vi "GoToKick.vi"(1 "goleiro?":bool, 3 "balls":T3[](array[typedef]), 4 "Robot in in":T4, 5 "atacando contra?":bool, 6 "Field Size in":T2, 7 "Target":dbl[](array[numeric]), 8 "Defender":bool, 9 "D ball - robot":dbl, 10 "AI Parameters":T1={"GotoKick"={"Dist do cone a frente"=150.0, "attacker farback"=1500.0, "Perto"=300.0, "min dist to kick"=150.0, "kick eps"=0.05, "Time to transition"=0.0}, "Attacker"={"CC chute"=0.09, "CC passe"=0.045, "Kick Force"=100.0, "D ball-robot Kick"=200.0, "D ball-robot Pass"=0.3}, "Defender"={"D max"=1700.0, "Vel p/ robô av"=1000.0, "Kick Force"=100.0, "D atk-def"=0.0, "D farback"=0.0}, "Timeout"={"Field/v in x"=6.0, "Dist Robots"=300, "Dist up in y"=300}, "Pose Striker"={"dist"=200.0, "Numeric"=-4.0, "dist 2"=200.0}, "Dist Stop"=300.0, "Distance when ball out"=200, "D central gap "=150.0, "T pass"=0.0, "Force ++"=0.0, "range kick"=0.0, "Chute alto"=TRUE, "Marcador novo"=TRUE} {"D central gap" format="%#_13g"; "Dist Stop" format="%#_13g"; "Pose Striker"."Numeric" format="%#_13g"; "Defender"."Kick Force" format="%#_13g"; "Defender"."Vel p/ robô av" format="%#_13g"; "Attacker"."D ball-robot Kick" format="%#_13g"; "Attacker"."Kick Force" format="%#_13g"; "Attacker"."CC passe" format="%#_13g"; "Attacker"."CC chute" format="%#_13g"; "GotoKick"."kick eps" format="%#_13g"; "GotoKick"."min dist to kick" format="%#_13g"; "GotoKick"."Perto" format="%#_13g"; "GotoKick"."attacker farback" format="%#_13g"; "GotoKick"."Dist do cone a frente" format="%#_13g"}, 11 "Cone de chute":dbl=0.09 format="%#_13g", 13 "Passe":bool, 18 "Kick Force":dbl=5.0 format="%#_13g", 19 "IA State Input in":T9) -> (0 "Current States":T6, 12 "Next State":T6, 14 "Robot out":T4, 17 "kick error":dbl)   [LabVIEW 2017]
uses:
  Core/AI Input.ctl
  Core/AI Robot.ctl
  Functions Enum.ctl
  AttackerStates.ctl
  Path Planning/RRT/PathDests.ctl
  Path Planning/RRT/PathDest.ctl
  Core/AI Ball.ctl
  Core/Field Size.ctl
  Core/AI Judge.ctl
  Command Enum.ctl
  Util/Events/Events.ctl
  AI Parameters.ctl
  <vilib>/Analysis/_algsub.llb/Real Vector Norm.vi
  <vilib>/Analysis/baseanly.llb/Real Dot Product.vi
  <vilib>/Analysis/coordinate.llb/2D Cartesian Coordinate Rotation (Scalar).vi
  <vilib>/Analysis/NI_AALPro.lvlib
  <vilib>/Analysis/NI_AALBase.lvlib
panel:
  out "Elapsed Time (s)":dbl
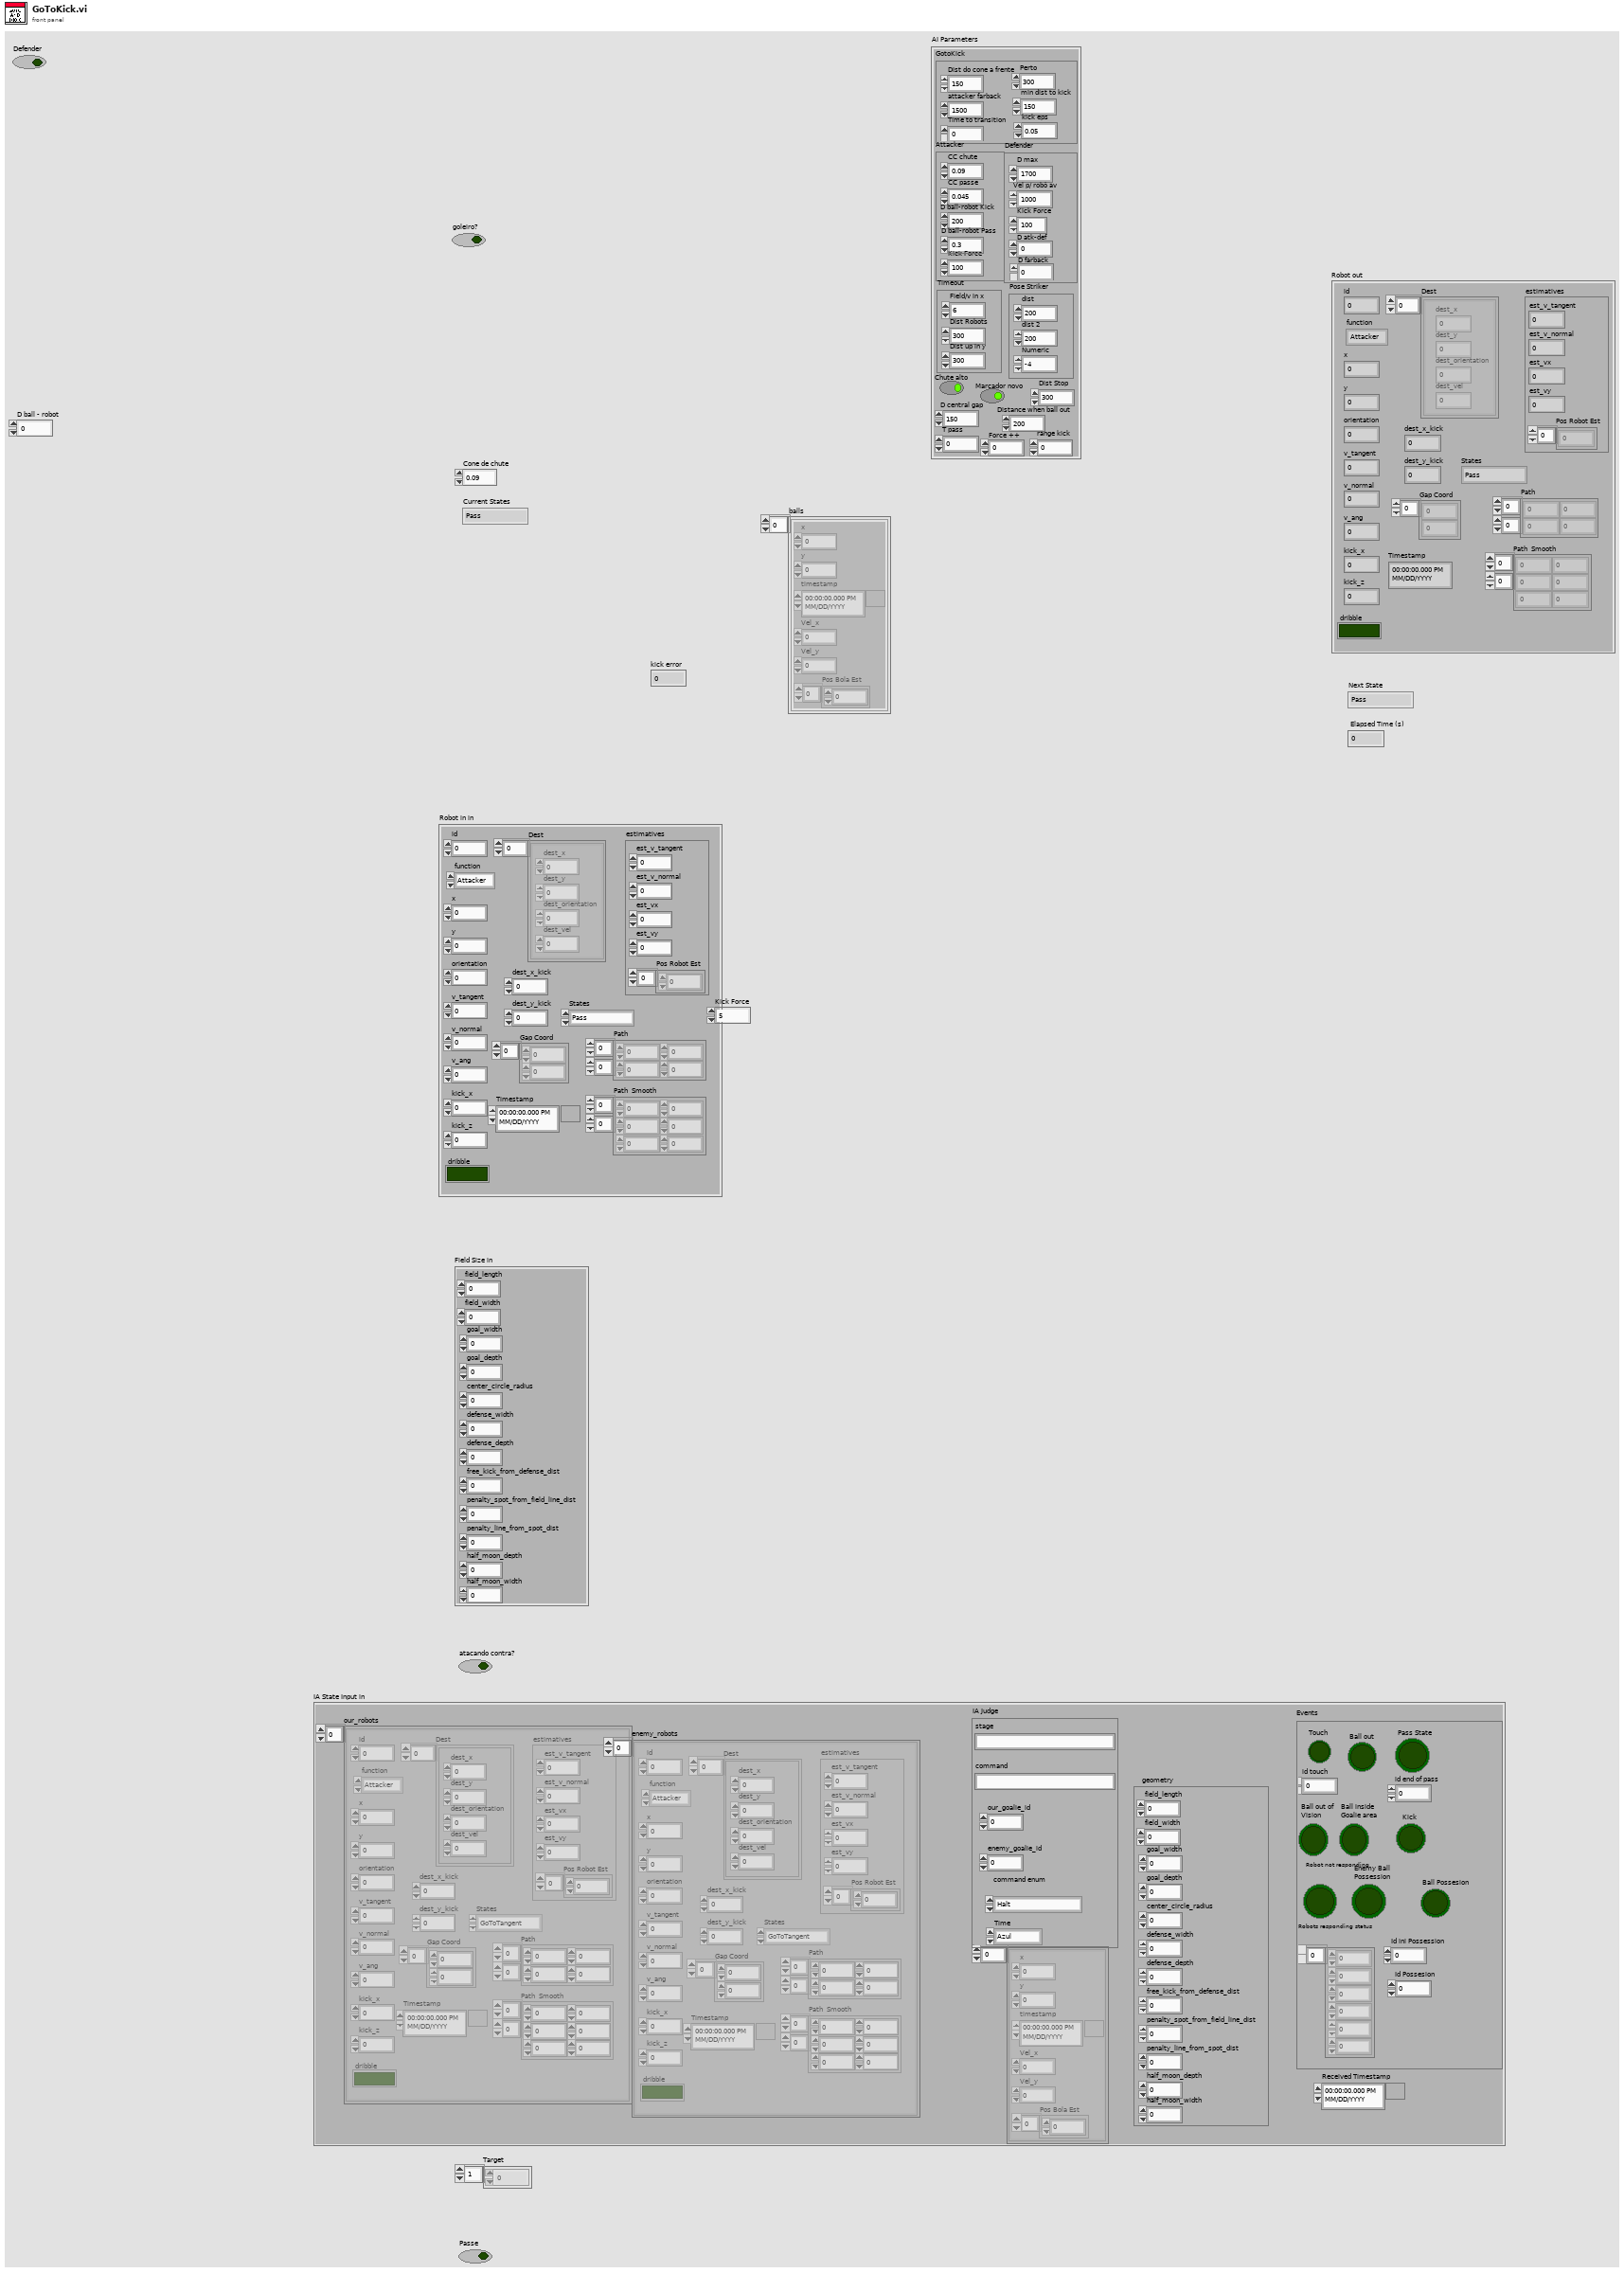
[diagram p1: front panel]
types:
  T1 = typedef "AI Parameters.ctl" = cluster{"GotoKick":cluster{"Dist do cone a frente":dbl, "attacker farback":dbl, "Perto":dbl, "min dist to kick":dbl, "kick eps":dbl, "Time to transition":dbl}, "Attacker":cluster{"CC chute":dbl, "CC passe":dbl, "Kick Force":dbl, "D ball-robot Kick":dbl, "D ball-robot Pass":dbl}, "Defender":cluster{"D max":dbl, "Vel p/ robô av":dbl, "Kick Force":dbl, "D atk-def":dbl, "D farback":dbl}, "Timeout":cluster{"Field/v in x":dbl, "Dist Robots":u32, "Dist up in y":u32}, "Pose Striker":cluster{"dist":dbl, "Numeric":dbl, "dist 2":dbl}, "Dist Stop":dbl, "Distance when ball out":i32, "D central gap ":dbl, "T pass":dbl, "Force ++":dbl, "range kick":dbl, "Chute alto":bool, "Marcador novo":bool}
  T2 = typedef "Field Size.ctl" = cluster{"field_length":u32, "field_width":u32, "goal_width":u32, "goal_depth":u32, "center_circle_radius":u32, "defense_width":u32, "defense_depth":u32, "free_kick_from_defense_dist":u32, "penalty_spot_from_field_line_dist":u32, "penalty_line_from_spot_dist":u32, "half_moon_depth":u32, "half_moon_width":u32}
  T3 = typedef "AI Ball.ctl" = cluster{"x":dbl, "y":dbl, "timestamp":timestamp, "Vel_x":dbl, "Vel_y":dbl, "Pos Bola Est":dbl[]}
  T4 = typedef "AI Robot.ctl" = cluster{"id":u32, "function":T5, "x":dbl, "y":dbl, "orientation":dbl, "v_tangent":dbl, "v_normal":dbl, "v_ang":dbl, "kick_x":dbl, "kick_z":dbl, "dribble":bool, "Timestamp":timestamp, "estimatives":cluster{"est_v_tangent":dbl, "est_v_normal":dbl, "est_vx":dbl, "est_vy":dbl, "Pos Robot Est":dbl[]}, "dest_x_kick":dbl, "dest_y_kick":dbl, "Gap Coord":dbl[], "States":T6, "Path ":dbl[][], "Path  Smooth":dbl[][], "Dest":T7}
  T5 = typedef "Functions Enum.ctl" = enum16{"Attacker", "Goalie", "Defender", "Striker", "Goto 0", "Dummy", "Kicker", "ZigZag"}
  T6 = typedef "AttackerStates.ctl" = enum16{"Pass", "GoToTangent", "BallGetting", "GoToKick", ""}
  T7 = typedef "PathDests.ctl" = T8[]
  T8 = typedef "PathDest.ctl" = cluster{"dest_x":dbl, "dest_y":dbl, "dest_orientation":dbl, "dest_vel":dbl}
  T9 = typedef "AI Input.ctl" = cluster{"our_robots":T4[], "enemy_robots":T4[], "balls":T3[], "geometry":T2, "IA Judge":T10, "Received Timestamp":timestamp, "Events":T12}
  T10 = typedef "AI Judge.ctl" = cluster{"stage":string, "command":string, "our_goalie_id":dbl, "enemy_goalie_id":dbl, "command enum":T11, "Time":enum16{"Azul", "Amarelo"}}
  T11 = typedef "Command Enum.ctl" = enum16{"Halt", "Stop", "Force Start", "PKA Normal Start", "Prepare Kickoff Ally", "PKE Normal Start", "Prepare Kickoff Enemy", "Prepare Penalty Ally", "PPA Normal Start", "Prepare Penalty Enemy", "PPE Normal Start", "Direct Free Enemy", "Direct Free Ally", "Indirect Free Enemy", "Indirect Free Ally", "Timeout Enemy", "Timeout Ally", "Goal Enemy", "Goal Ally", "Ball Placement Enemy", "Ball Placement Ally", "Normal Half Time", "Extra Time Break", "Extra Half Time", "None", "Post Game"}
  T12 = typedef "Events.ctl" = cluster{"Touch":bool, "Ball out":bool, "id touch":dbl, "Ball out of \nVision":bool, "Ball inside \nGoalie area":bool, "Robot not responding":bool, "Robots responding status":dbl[], "Enemy Ball \nPossession":bool, "Pass State":bool, "id end of pass":dbl, "Kick":bool, "Id ini Possession":dbl, "Ball Possesion":bool, "Id Possesion":dbl}
  T13 = cluster{"Dist do cone a frente":dbl, "attacker farback":dbl, "Perto":dbl, "min dist to kick":dbl, "kick eps":dbl, "Time to transition":dbl}
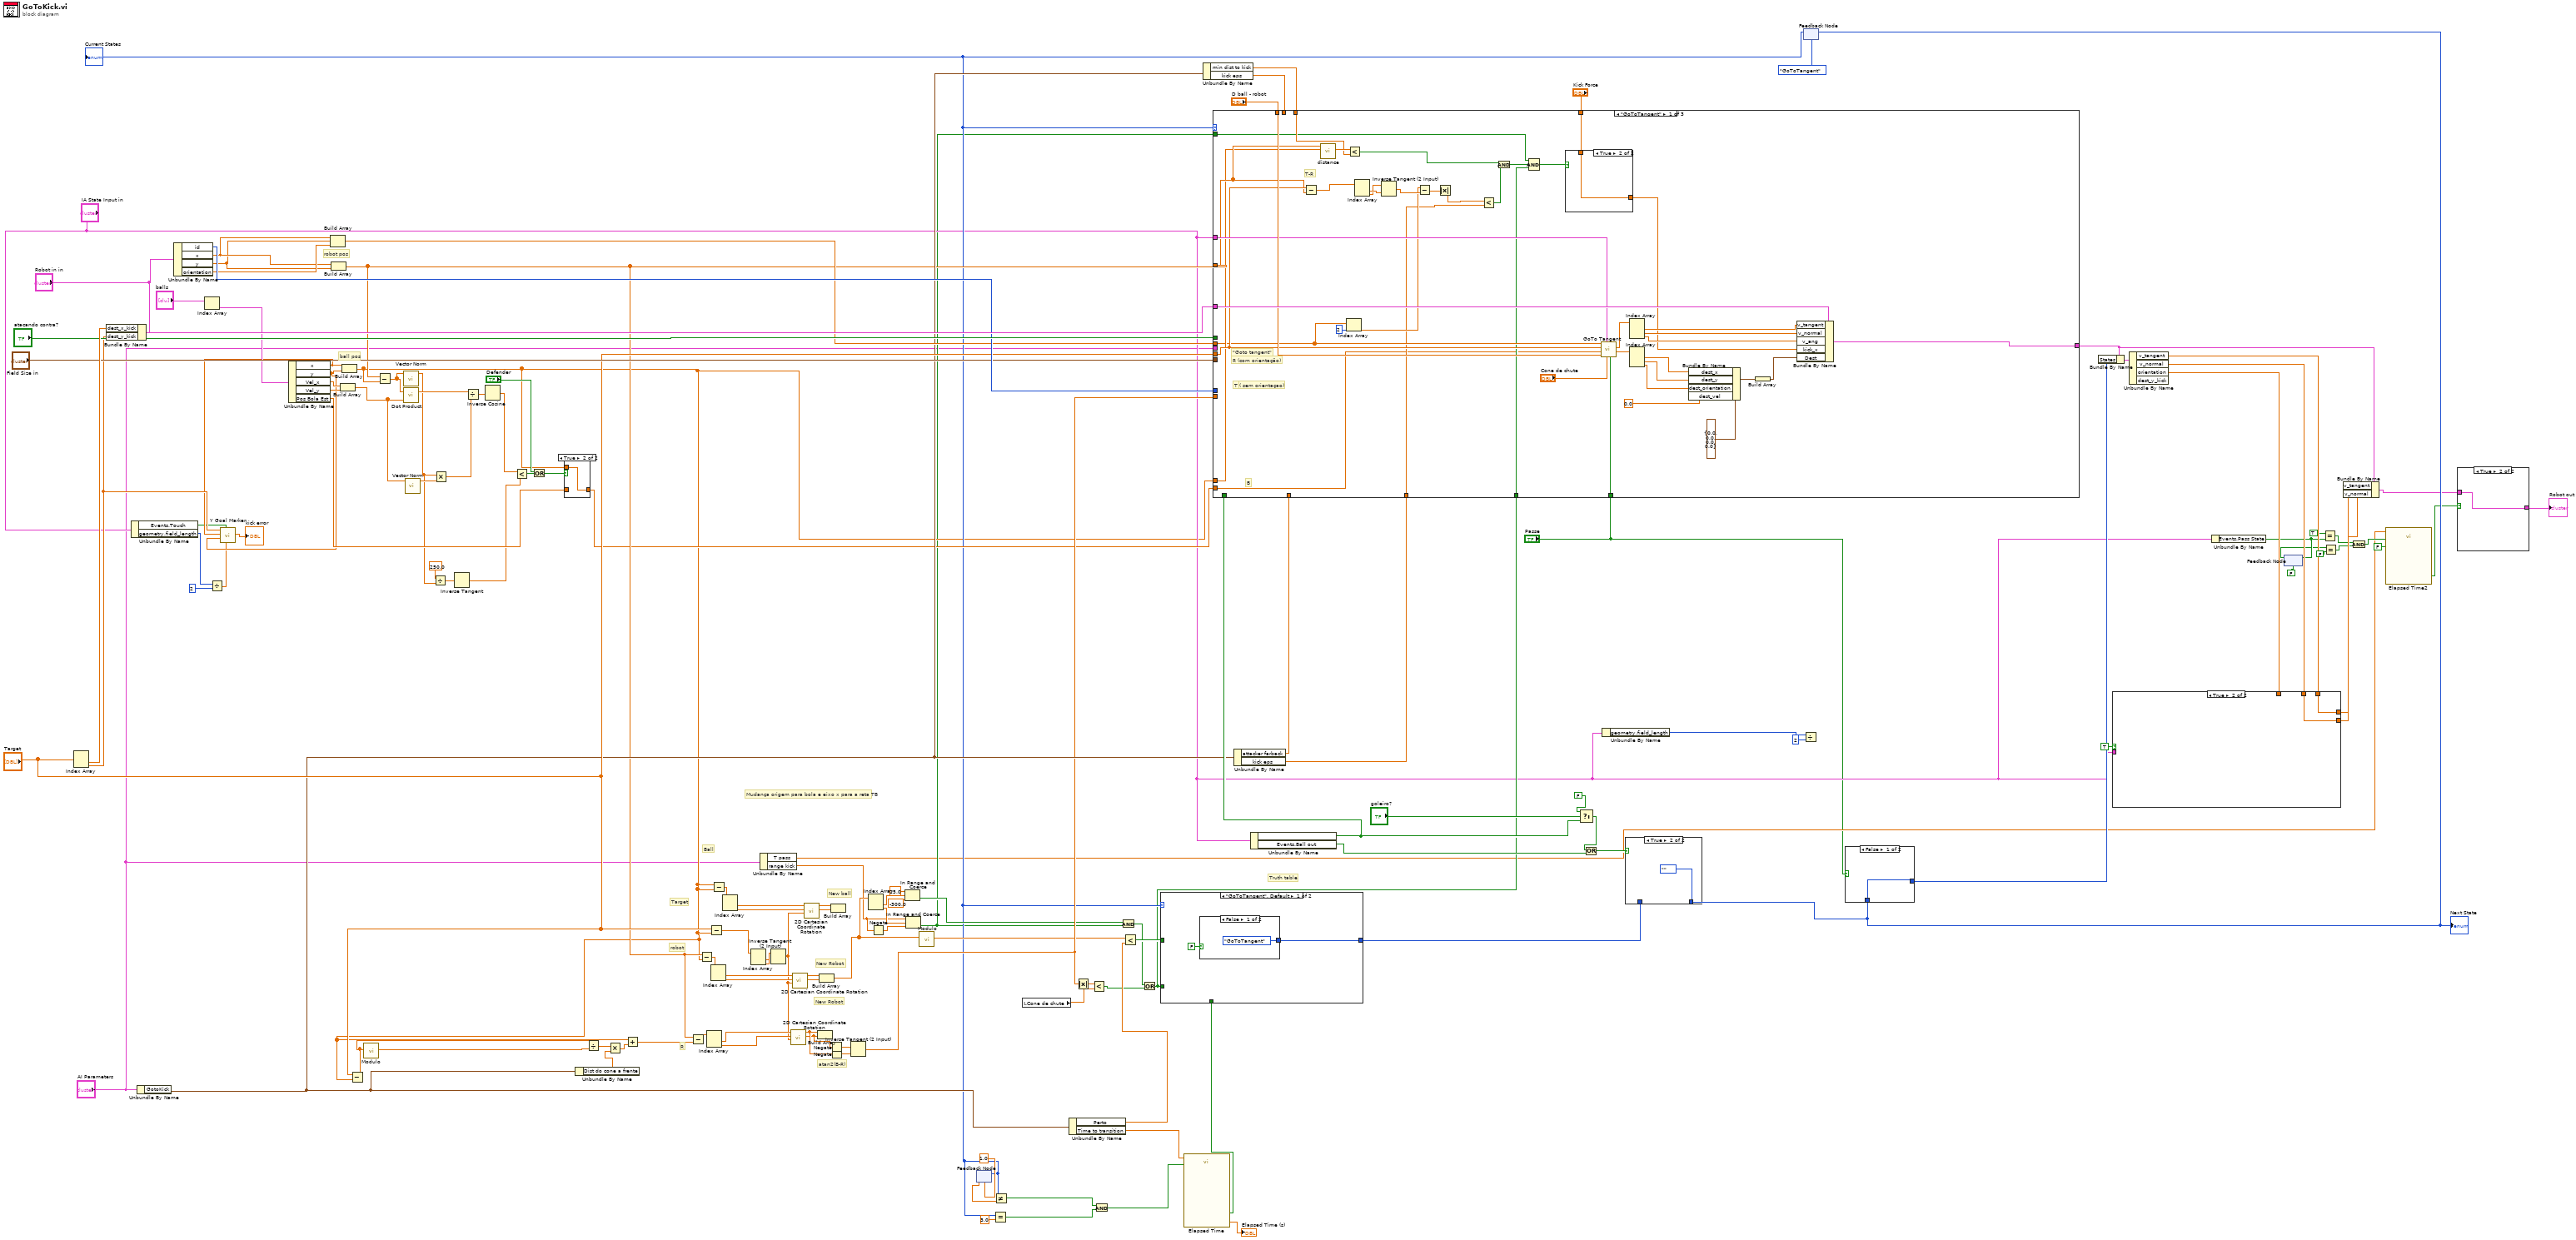
[diagram p0: block diagram]
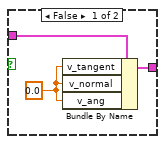
[diagram p2: hidden frame]
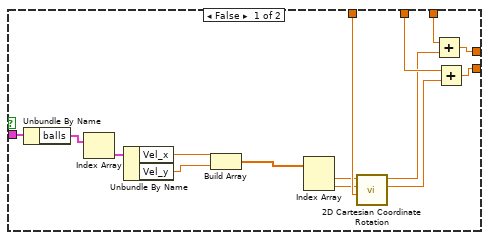
[diagram p3: hidden frame]
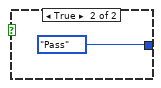
[diagram p5: hidden frame]
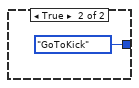
[diagram p6: hidden frame]
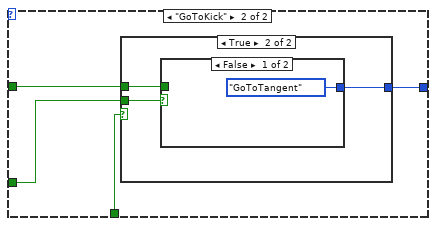
[diagram p7: hidden frame]
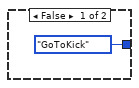
[diagram p8: hidden frame]
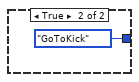
[diagram p9: hidden frame]
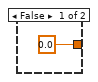
[diagram p11: hidden frame]
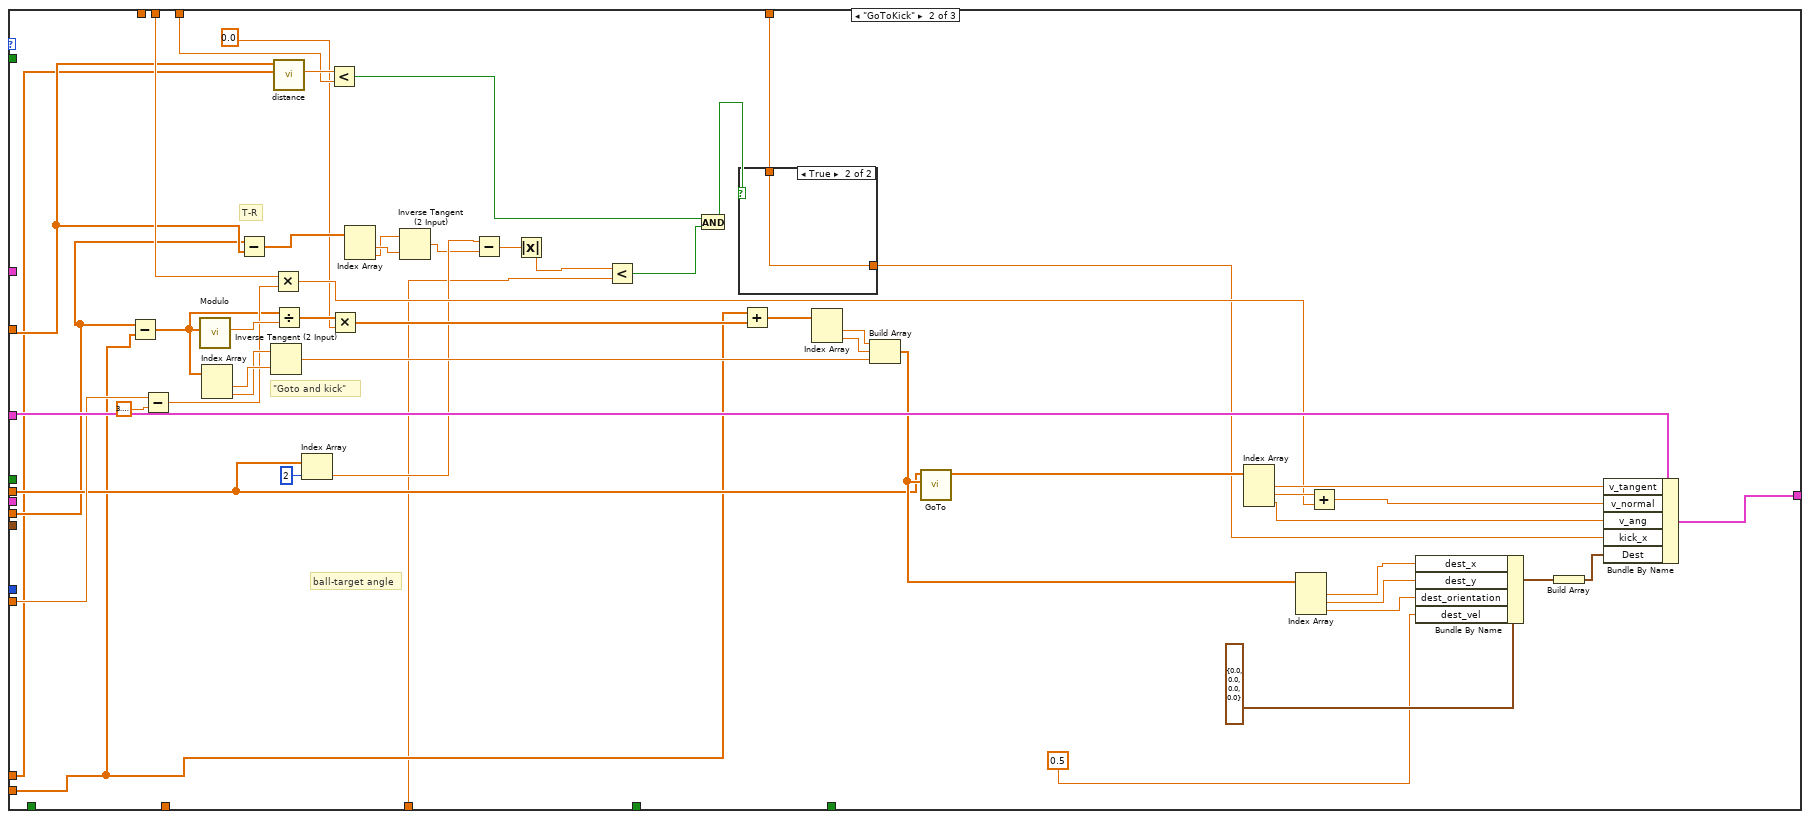
[diagram p12: hidden frame]
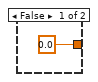
[diagram p13: hidden frame]
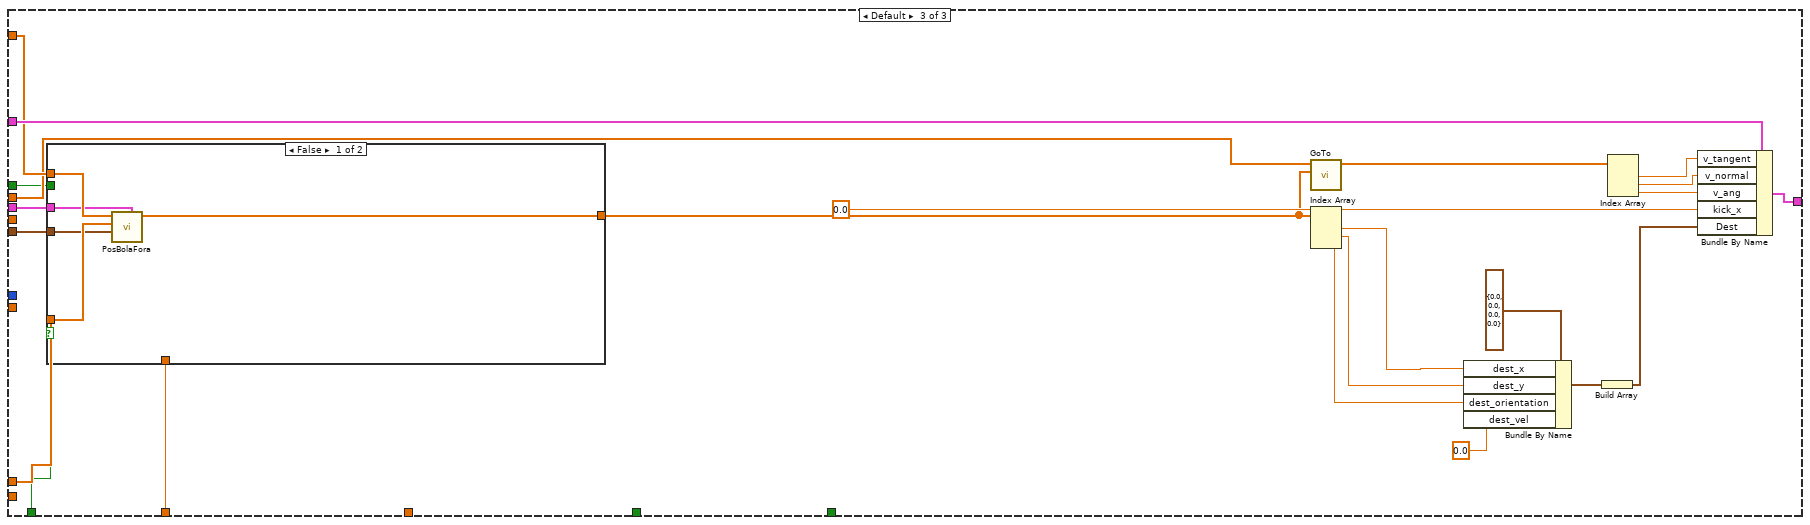
[diagram p14: hidden frame]
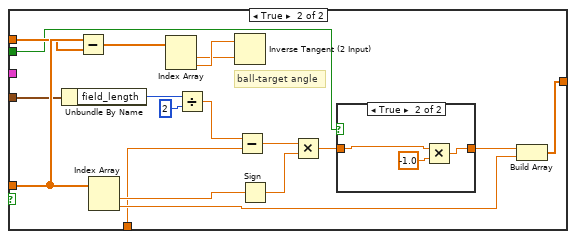
[diagram p15: hidden frame]
diagram:
  # "New ball"
  # "robot"
  # "atan2(B-R)"
  # "New Robot"
  # "New Robot"
  # "R"
  # "Ball"
  # "Target"
  # "Mudança origem para bola e eixo x para a reta TB"
  # "Truth table"
  # "robot pos"
  # "ball pos"
  n1 = Index Array(array="Target") -> (element #1=w139:dbl, element #2=w34:dbl)  [unwired: 2 in]
  n2 = Bundle By Name(cluster="Robot in in", "dest_x_kick"=w139, "dest_y_kick"=w34) -> (w135:T4)
  n3 = Unbundle By Name("IA State Input in") -> ("Events.Touch"=w30:bool, "geometry.field_length"=w29:u32)
  n4 = Unbundle By Name("AI Parameters") -> ("GotoKick"=w80:T13)
  n5 = Unbundle By Name("Robot in in") -> ("id"=w110:u32, "x"=w74:dbl, "y"=w73:dbl, "orientation"=w101:dbl)
  n6 = Index Array(array="balls") -> (element=w99:T3)  [unwired: 1 in]
  n7 = Divide(x=w29, y=u32 2) -> (x/y=w27:dbl)
  n8 = Unbundle By Name(w99) -> ("x"=w33:dbl, "y"=w32:dbl, "Vel_x"=w56:dbl, "Vel_y"=w55:dbl, "Pos Bola Est"=w47:dbl[])
  n9 = call "Y Goal Marker.vi"("goal x"=w27, "Touch"=w30, "y"=w32, "x"=w33, "dest_y_kick"=w34) -> ("kick error"=→"kick error":dbl)  [unwired: 6 in]
  n10 = Build Array(w74, w73, w101) -> (w100:dbl[])
  n11 = Build Array(w74, w73) -> (w57:dbl[])
  n12 = Build Array(w56, w55) -> (w53:dbl[])
  n13 = Build Array(w33, w32) -> (w20:dbl[])
  n14 = Subtract(x="Target", y=w20) -> (x-y=w129:dbl[])
  n15 = call "Modulo.vi"("2D vector"=w129) -> ("Modulo"=w128:dbl)  [unwired: 10 in]
  n16 = Subtract(x=w57, y=w20) -> (x-y=w54:dbl[])
  n17 = call-poly <vilib>:"Dot Product.vi"("Y Vector"=w53, "X Vector"=w54) -> ("X * Y"=w50:dbl)  [unwired: 1 out]
  n18 = call-poly <vilib>:"Vector Norm.vi"("Input Vector"=w54) -> ("norm"=w44:dbl)  [unwired: 9 in, 1 out]
  n19 = call-poly <vilib>:"Vector Norm.vi"("Input Vector"=w53) -> ("norm"=w52:dbl)  [unwired: 9 in, 1 out]
  n20 = Divide(x=250.0, y=w44) -> (x/y=w45:dbl)
  n21 = Multiply(x=w44, y=w52) -> (x*y=w51:dbl)
  n22 = Inverse Tangent(1:w45) -> (0:w42:dbl)
  n23 = Divide(x=w50, y=w51) -> (x/y=w49:dbl)
  n24 = Inverse Cosine(1:w49) -> (0:w48:dbl)
  n25 = Less?(x=w48, y=w42) -> (x < y?=w22:bool)
  n26 = Or(x="Defender", y=w22) -> (x .or. y?=w23:bool)
  n27 = case shown="True" w23 {
    tunnel: w47 -> [w140 _]
    tunnel: [w140 w141] -> w46
    tunnel: w20 -> [_ w141]
    frame False {
    }
    frame True {
    }
  }
  n28 = Unbundle By Name(w80) -> ("Dist do cone a frente"=w86:dbl)
  n29 = Divide(x=w129, y=w128) -> (x/y=w127:dbl[])
  n30 = Multiply(x=w127, y=w86) -> (x*y=w126:dbl[])
  n31 = Add(x=w20, y=w126) -> (x+y=w130:dbl[])
  n32 = Subtract(x=w57, y=w130) -> (x-y=w131:dbl[])
  n33 = Subtract(x=w57, y=w20) -> (x-y=w104:dbl[])
  n34 = Index Array(array=w131) -> (element #1=w132:dbl, element #2=w133:dbl)  [unwired: 2 in]
  n35 = Subtract(x="Target", y=w20) -> (x-y=w105:dbl[])
  n36 = Index Array(array=w104) -> (element #1=w102:dbl, element #2=w103:dbl)  [unwired: 2 in]
  n37 = Subtract(x=w20, y=w20) -> (x-y=w70:dbl[])
  n38 = Index Array(array=w70) -> (element #1=w68:dbl, element #2=w69:dbl)  [unwired: 2 in]
  n39 = Index Array(array=w105) -> (element #1=w106:dbl, element #2=w107:dbl)  [unwired: 2 in]
  n40 = Unbundle By Name("AI Parameters") -> ("T pass"=w2:dbl, "range kick"=w3:dbl)
  n41 = Inverse Tangent (2 Input)(1:w106, 2:w107) -> (0:w67:dbl)
  n42 = call-poly <vilib>:"2D Cartesian Coordinate Rotation.vi"("theta"=w67, "y"=w133, "x"=w132) -> ("y out"=w124:dbl, "x out"=w125:dbl)  [unwired: 6 in, 1 out]
  n43 = call-poly <vilib>:"2D Cartesian Coordinate Rotation.vi"("theta"=w67, "y"=w103, "x"=w102) -> ("y out"=w109:dbl, "x out"=w66:dbl)  [unwired: 6 in, 1 out]
  n44 = call-poly <vilib>:"2D Cartesian Coordinate Rotation.vi"("theta"=w67, "y"=w69, "x"=w68) -> ("y out"=w71:dbl, "x out"=w72:dbl)  [unwired: 6 in, 1 out]
  n45 = Build Array(w125, w124) -> ()  [unwired: 1 out]
  n46 = Build Array(w66, w109) -> (w65:dbl[])
  n47 = Negate(x=w124) -> (-x=w122:dbl)
  n48 = Negate(x=w125) -> (-x=w123:dbl)
  n49 = Build Array(w72, w71) -> ()  [unwired: 1 out]
  n50 = Inverse Tangent (2 Input)(1:w123, 2:w122) -> (0:w78:dbl)
  n51 = Index Array(array=w65) -> (element #1=w64:dbl, element #2=w63:dbl)  [unwired: 2 in]
  n52 = Negate(x=w3) -> (-x=w4:dbl)
  n53 = In Range and Coerce(upper limit=25.0, x=w64, lower limit=-300.0) -> (In Range?=w60:bool)  [unwired: 1 out]
  n54 = In Range and Coerce(upper limit=w3, x=w63, lower limit=w4) -> (In Range?=w6:bool)  [unwired: 1 out]
  n55 = call "Modulo.vi"("2D vector"=w65) -> ("Modulo"=w77:dbl)  [unwired: 10 in]
  n56 = feedback #1(1.0 ("Current State")) -> (w116:dbl)
  n57 = local read "Cone de chute"() -> (w25:dbl)
  n58 = Unbundle By Name(w80) -> ("Perto"=w76:dbl, "Time to transition"=w82:dbl)
  n59 = Absolute Value(x=w78) -> (abs(x)=w79:dbl)
  n60 = Less?(x=w79, y=w25) -> (x < y?=w59:bool)
  n61 = And(x=w60, y=w6) -> (x .and. y?=w58:bool)
  n62 = Less?(x=w77, y=w76) -> (x < y?=w75:bool)
  n63 = Or(x=w58, y=w59) -> (x .or. y?=w39:bool)
  n64 = Unbundle By Name(w80) -> ("min dist to kick"=w84:dbl, "kick eps"=w83:dbl)
  n65 = Unbundle By Name(w80) -> ("attacker farback"=w85:dbl, "kick eps"=w35:dbl)
  n66 = Unbundle By Name("IA State Input in") -> ("Events.Ball inside \nGoalie area"=w88:bool, "Events.Ball out"=w120:bool)
  n67 = Select(t=FALSE, s="goleiro?", f=w88) -> (s? t:f=w87:bool)
  n68 = Or(x=w87, y=w120) -> (x .or. y?=w121:bool)
  n69 = Unbundle By Name("IA State Input in") -> ("geometry.field_length"=w37:u32)
  n70 = Divide(x=w37, y=u32 2) -> ()  [unwired: 1 out]
  n71 = feedback #2(AttackerStates."GoToTangent" ("Next State")) -> (w41:T6)
  "Current States" <- w41
  n72 = feedback-in #1(w41) -> ()
  n73 = Equal?(x=w41, y=3.0) -> (x = y?=w113:bool)
  n74 = Not Equal?(x=w41, y=w116) -> (x != y?=w114:bool)
  n75 = And(x=w114, y=w113) -> (x .and. y?=w118:bool)
  n76 = call "Elapsed Time"("Time Target (s)"=w82, "Reset"=w118) -> ("Elapsed Time (s)"=→"Elapsed Time (s)":dbl, "Time has Elapsed"=w111:bool)  [unwired: 10 in, 6 out]
  n77 = case shown="\"GoToTangent\", Default" w41 {
    tunnel: [w143 w148] -> w136
    tunnel: w111 -> [_ w149]
    tunnel: w39 -> [_ w147]
    tunnel: w75 -> [_ w146]
    frame "GoToTangent", Default {
      n78 = case shown="False" FALSE {
        tunnel: [AttackerStates."GoToTangent" ("Next State") AttackerStates."GoToKick" ("Next State")] -> w143
        frame False {
        }
        frame True {
        }
      }
    }
    frame "GoToKick" {
      n79 = case shown="True" w149 {
        tunnel: [AttackerStates."GoToKick" ("Next State") w153] -> w148
        tunnel: w147 -> [_ w152]
        tunnel: w146 -> [_ w151]
        frame False {
        }
        frame True {
          n80 = case shown="False" w152 {
            tunnel: [AttackerStates."GoToTangent" ("Next State") AttackerStates."GoToKick" ("Next State")] -> w153
            tunnel: w151 -> [_ _]
            frame False {
            }
            frame True {
            }
          }
        }
      }
    }
  }
  n81 = case shown="\"GoToTangent\"" w41 {
    tunnel: [w191 w251 w276] -> w38
    tunnel: w135 -> [w192 w250 w275]
    tunnel: w100 -> [w173 w220 w269]
    tunnel: w57 -> [w177 w214 w271]
    tunnel: w20 -> [w176 w210 w272]
    tunnel: "Target" -> [w178 w213 _]
    tunnel: "Field Size in" -> [_ _ w270]
    tunnel: w110 -> [_ _ _]
    tunnel: w88 -> [_ _ w266]
    tunnel: "atacando contra?" -> [_ _ w265]
    tunnel: w78 -> [_ w233 _]
    tunnel: w85 -> [_ _ w262]
    tunnel: w84 -> [w175 w228 _]
    tunnel: w83 -> [_ w227 _]
    tunnel: "D ball - robot" -> [w190 _ _]
    tunnel: "AI Parameters" -> [_ _ w261]
    tunnel: "IA State Input in" -> [w189 _ _]
    tunnel: w46 -> [w165 w211 _]
    tunnel: "Kick Force" -> [w179 w209 _]
    tunnel: w39 -> [w169 _ _]
    tunnel: w35 -> [w167 w208 _]
    tunnel: w6 -> [w164 _ _]
    tunnel: "Passe" -> [w163 _ _]
    frame "GoToTangent" {
      # "T-R"
      # "\"Goto tangent\""
      # "B"
      # "T"
      # "R ( sem orientaçao)"
      # "R (com orientação)"
      n82 = Subtract(x=w178, y=w177) -> (x-y=w185:dbl[])
      n83 = call "distance.vi"("target pos"=w176, "obj pos"=w177) -> ("sqrt(x)"=w188:dbl)  [unwired: 9 in]
      n84 = Index Array(array=w173, index=2) -> (element=w172:dbl)
      n85 = Less?(x=w188, y=w175) -> (x < y?=w184:bool)
      n86 = Index Array(array=w185) -> (element #1=w187:dbl, element #2=w186:dbl)  [unwired: 2 in]
      n87 = Inverse Tangent (2 Input)(1:w187, 2:w186) -> (0:w183:dbl)
      n88 = Subtract(x=w172, y=w183) -> (x-y=w182:dbl)
      n89 = Absolute Value(x=w182) -> (abs(x)=w180:dbl)
      n90 = Less?(x=w180, y=w167) -> (x < y?=w181:bool)
      n91 = And(x=w184, y=w181) -> (x .and. y?=w170:bool)
      n92 = Compound Arithmetic op=AND(w164, w170, w169) -> (w168:bool)
      n93 = case shown="True" w168 {
        tunnel: [0.0 w199] -> w171
        tunnel: w179 -> [_ w199]
        frame False {
        }
        frame True {
        }
      }
      n94 = call "GoTo Tangent.vi"("Passe"=w163, "Cone de chute"="Cone de chute", "IA State Input in"=w189, "distance between ball and robot"=w190, "Ball"=w165, "Target"=w178, "R"=w173) -> ("Destination"=w194:dbl[], "Output\nVelocity"=w195:dbl[])  [unwired: 3 in]
      n95 = Index Array(array=w195) -> (element #1=w197:dbl, element #2=w193:dbl, element #3=w196:dbl)  [unwired: 3 in]
      n96 = Index Array(array=w194) -> (element #1=w158:dbl, element #2=w157:dbl, element #3=w156:dbl)  [unwired: 3 in]
      n97 = Bundle By Name(cluster=T8 {"dest_x"=0.0, "dest_y"=0.0, "dest_orientation"=0.0, "dest_vel"=0.0} ("Dest"), "dest_x"=w158, "dest_y"=w157, "dest_orientation"=w156, "dest_vel"=0.0) -> (w161:T8)
      n98 = Build Array(w161) -> (w159:T8[])
      n99 = Bundle By Name(cluster=w192, "v_tangent"=w197, "v_normal"=w193, "v_ang"=w196, "kick_x"=w171, "Dest"=w159) -> (w191:T4)
    }
    frame "GoToKick" {
      # "T-R"
      # "ball-target angle"
      # "\"Goto and kick\""
      n100 = Subtract(x=w213, y=w211) -> (x-y=w224:dbl[])
      n101 = Subtract(x=w233, y=3.141592653589793) -> (x-y=w231:dbl)
      n102 = call "Modulo.vi"("2D vector"=w224) -> ("Modulo"=w238:dbl)  [unwired: 10 in]
      n103 = Index Array(array=w224) -> (element #1=w248:dbl, element #2=w247:dbl)  [unwired: 2 in]
      n104 = Subtract(x=w213, y=w214) -> (x-y=w223:dbl[])
      n105 = Inverse Tangent (2 Input)(1:w248, 2:w247) -> (0:w246:dbl)
      n106 = Multiply(x=w227, y=w231) -> (x*y=w234:dbl)
      n107 = call "distance.vi"("target pos"=w210, "obj pos"=w214) -> ("sqrt(x)"=w249:dbl)  [unwired: 9 in]
      n108 = Divide(x=w224, y=w238) -> (x/y=w239:dbl[])
      n109 = Index Array(array=w220, index=2) -> (element=w218:dbl)
      n110 = Less?(x=w249, y=w228) -> (x < y?=w222:bool)
      n111 = Multiply(x=w239, y=0.0) -> (x*y=w241:dbl[])
      n112 = Index Array(array=w223) -> (element #1=w226:dbl, element #2=w225:dbl)  [unwired: 2 in]
      n113 = Inverse Tangent (2 Input)(1:w226, 2:w225) -> (0:w217:dbl)
      n114 = Subtract(x=w218, y=w217) -> (x-y=w216:dbl)
      n115 = Absolute Value(x=w216) -> (abs(x)=w212:dbl)
      n116 = Less?(x=w212, y=w208) -> (x < y?=w215:bool)
      n117 = And(x=w222, y=w215) -> (x .and. y?=w221:bool)
      n118 = case shown="True" w221 {
        tunnel: [0.0 w253] -> w230
        tunnel: w209 -> [_ w253]
        frame False {
        }
        frame True {
        }
      }
      n119 = Add(x=w211, y=w241) -> (x+y=w240:dbl[])
      n120 = Index Array(array=w240) -> (element #1=w245:dbl, element #2=w244:dbl)  [unwired: 2 in]
      n121 = Build Array(w245, w244, w246) -> (w237:dbl[])
      n122 = call "GoTo.vi"("Target"=w237, "Position"=w220) -> ("Output\nVelocity"=w243:dbl[])  [unwired: 8 in, 1 out]
      n123 = Index Array(array=w243) -> (element #1=w242:dbl, element #2=w236:dbl, element #3=w229:dbl)  [unwired: 3 in]
      n124 = Index Array(array=w237) -> (element #1=w203:dbl, element #2=w202:dbl, element #3=w201:dbl)  [unwired: 3 in]
      n125 = Add(x=w236, y=w234) -> (x+y=w235:dbl)
      n126 = Bundle By Name(cluster=T8 {"dest_x"=0.0, "dest_y"=0.0, "dest_orientation"=0.0, "dest_vel"=0.0} ("Dest"), "dest_x"=w203, "dest_y"=w202, "dest_orientation"=w201, "dest_vel"=0.5) -> (w205:T8)
      n127 = Build Array(w205) -> (w204:T8[])
      n128 = Bundle By Name(cluster=w250, "v_tangent"=w242, "v_normal"=w235, "v_ang"=w229, "kick_x"=w230, "Dest"=w204) -> (w251:T4)
    }
    frame Default {
      n129 = case shown="False" w266 {
        tunnel: w272 -> [w281 w293]
        tunnel: w271 -> [w280 w291]
        tunnel: w270 -> [w279 w292]
        tunnel: [w278 w298] -> w267
        tunnel: w265 -> [_ w287]
        tunnel: w262 -> [_ w282]
        tunnel: w261 -> [w277 _]
        frame False {
          n130 = call "PosBolaFora.vi"("AI Parameters"=w277, "Field Size in"=w279, "Position da bola"=w281, "Position do robot"=w280) -> ("Target"=w278:dbl[])  [unwired: 7 in]
        }
        frame True {
          # "ball-target angle"
          n131 = Unbundle By Name(w292) -> ("field_length"=w290:u32)
          n132 = Subtract(x=w293, y=w291) -> (x-y=w296:dbl[])
          n133 = Index Array(array=w293) -> (element #1=w286:dbl, element #2=w299:dbl)  [unwired: 2 in]
          n134 = Index Array(array=w296) -> (element #1=w294:dbl, element #2=w295:dbl)  [unwired: 2 in]
          n135 = Divide(x=w290, y=u32 2) -> (x/y=w288:dbl)
          n136 = Inverse Tangent (2 Input)(1:w294, 2:w295) -> ()  [unwired: 1 out]
          n137 = Subtract(x=w288, y=w282) -> (x-y=w285:dbl)
          n138 = Sign(1:w286) -> (0:w284:dbl)
          n139 = Multiply(x=w285, y=w284) -> (x*y=w283:dbl)
          n140 = case shown="True" w287 {
            tunnel: w283 -> [w300 w303]
            tunnel: [w300 w302] -> w297
            frame False {
            }
            frame True {
              n141 = Multiply(x=w303, y=-1.0) -> (x*y=w302:dbl)
            }
          }
          n142 = Build Array(w297, w299) -> (w298:dbl[])
        }
      }
      n143 = call "GoTo.vi"("Target"=w267, "Position"=w269) -> ("Output\nVelocity"=w268:dbl[])  [unwired: 8 in, 1 out]
      n144 = Index Array(array=w267) -> (element #1=w256:dbl, element #2=w255:dbl, element #3=w254:dbl)  [unwired: 3 in]
      n145 = Bundle By Name(cluster=T8 {"dest_x"=0.0, "dest_y"=0.0, "dest_orientation"=0.0, "dest_vel"=0.0} ("Dest"), "dest_x"=w256, "dest_y"=w255, "dest_orientation"=w254, "dest_vel"=0.0) -> (w259:T8)
      n146 = Build Array(w259) -> (w257:T8[])
      n147 = Index Array(array=w268) -> (element #1=w273:dbl, element #2=w264:dbl, element #3=w263:dbl)  [unwired: 3 in]
      n148 = Bundle By Name(cluster=w275, "v_tangent"=w273, "v_normal"=w264, "v_ang"=w263, "kick_x"=0.0, "Dest"=w257) -> (w276:T4)
    }
  }
  n149 = case shown="True" w121 {
    tunnel: [w304 AttackerStates."" ("Next State")] -> w98
    tunnel: w136 -> [w304 _]
    frame False {
    }
    frame True {
    }
  }
  "Next State" <- w98
  n150 = feedback-in #2(w98) -> ()
  n151 = case shown="False" "Passe" {
    tunnel: w98 -> [w306 _]
    tunnel: [w306 AttackerStates."Pass" ("Next State")] -> w137
    frame False {
    }
    frame True {
    }
  }
  n152 = Bundle By Name(cluster=w38, "States"=w137) -> (w96:T4)
  n153 = Unbundle By Name(w96) -> ("v_tangent"=w94:dbl, "v_normal"=w93:dbl, "orientation"=w95:dbl)  [unwired: 1 out]
  n154 = case shown="True" TRUE {
    tunnel: w95 -> [w322 _]
    tunnel: w94 -> [w321 w324]
    tunnel: w93 -> [w320 w323]
    tunnel: [w319 w323] -> w92
    tunnel: [w318 w324] -> w91
    tunnel: "IA State Input in" -> [w317 _]
    frame False {
      n155 = Unbundle By Name(w317) -> ("balls"=w316:T3[])
      n156 = Index Array(array=w316) -> (element=w315:T3)  [unwired: 1 in]
      n157 = Unbundle By Name(w315) -> ("Vel_x"=w311:dbl, "Vel_y"=w310:dbl)
      n158 = Build Array(w311, w310) -> (w312:dbl[])
      n159 = Index Array(array=w312) -> (element #1=w314:dbl, element #2=w313:dbl)  [unwired: 2 in]
      n160 = call-poly <vilib>:"2D Cartesian Coordinate Rotation.vi"("theta"=w322, "y"=w313, "x"=w314) -> ("y out"=w308:dbl, "x out"=w309:dbl)  [unwired: 6 in, 1 out]
      n161 = Add(x=w321, y=w309) -> (x+y=w318:dbl)
      n162 = Add(x=w320, y=w308) -> (x+y=w319:dbl)
    }
    frame True {
    }
  }
  n163 = Unbundle By Name("IA State Input in") -> ("Events.Pass State"=w14:bool)
  n164 = feedback-in #3(w14) -> ()
  n165 = feedback #3(FALSE ("Pass State")) -> (w12:bool)
  n166 = Equal?(x=TRUE, y=w14) -> (x = y?=w9:bool)
  n167 = Equal?(x=w12, y=FALSE) -> (x = y?=w8:bool)
  n168 = Bundle By Name(cluster=w38, "v_tangent"=w91, "v_normal"=w92) -> (w18:T4)
  n169 = And(x=w9, y=w8) -> (x .and. y?=w7:bool)
  n170 = call "Elapsed Time2"("Time Target (s)"=w2, "Reset"=w7, "Auto Reset"=FALSE) -> ("Time has Elapsed"=w15:bool)  [unwired: 9 in, 7 out]
  n171 = case shown="True" w15 {
    tunnel: w18 -> [w327 w328]
    tunnel: [w326 w328] -> w17
    frame False {
      w325 = 0.0
      n172 = Bundle By Name(cluster=w327, "v_tangent"=w325, "v_normal"=w325, "v_ang"=w325) -> (w326:T4)
    }
    frame True {
    }
  }
  "Robot out" <- w17
